vi "SAOMM-OffsetGUI.vi"(0 "Hexapod VRN":refnum<visa-resource-name>="COM4", 1 "Active Refnum":refnum<vi>, 2 "PrAMS-ACK":refnum<vi>, 7 "output cluster":T1, 13 "MessageType":cluster{string[], u32[]}={["emtError", "emtAreYouThere", "emtAcknowledgment", "emtGetClientType", "emtClientType", "emtGetImageExposureTime", "emtSetImageExposureTime", "emtImageExposureTime", "emtGetOptimalExposureTime", "emtSetOptimalExposureTime", "emtOptimalExposureTime", "emtGetImageEMGain", "emtSetImageEMGain", "emtImageEMGain", "emtGetFPGACtrl", "emtSetFPGACtrl", "emtFPGACtrl", "emtGetImageWidth", "emtSetImageWidth", "emtImageWidth", "emtGetImageHeight", "emtSetImageHeight", "emtImageHeight", "emtGetImageBinning", "emtSetImageBinning", "emtImageBinning", "emtGetImageDisplayFrameRate", "emtSetImageDisplayFrameRate", "emtImageDisplayFrameRate", "emtGetROIWidth", "emtSetROIWidth", "emtROIWidth", "emtGetROIHeight", "emtSetROIHeight", "emtROIHeight", "emtGetROIXOffset", "emtSetROIXOffset", "emtROIXOffset", "emtGetROIYOffset", "emtSetROIYOffset", "emtROIYOffset", "emtStartAcquisition", "mtStopAcquisition", "emtAcquisitionStarted", "emtAcquisitionStopped", "emtGetFalconImage", "emtFalconImage"], [1, 2, 3, 4, 5, 1001, 1101, 1201, 1002, 1102, 1202, 1003, 1103, 1203, 1004, 1104, 1204, 1005, 1105, 1205, 1006, 1106, 1206, 1007, 1107, 1207, 1008, 1108, 1208, 1009, 1109, 1209, 1010, 1110, 1210, 1011, 1111, 1211, 1012, 1112, 1212, 1130, 1131, 1150, 1151, 1070, 1270]}) -> (8 "Error":bool)   [LabVIEW 2011]
uses:
  Polymorphics/Num2littleEndian(DBL).vi
panel:
  in  "Signature":u32=1886544237
  in  "Cancel":bool
  in  "Send":bool
  in  "X":dbl caption="Pos" format="%.4f"
  in  "Y":dbl caption="Pos" format="%.4f"
  in  "Z":dbl caption="Pos" format="%.4f"
  in  "U":dbl caption="Pos" format="%.4f"
  in  "V":dbl caption="Pos" format="%.4f"
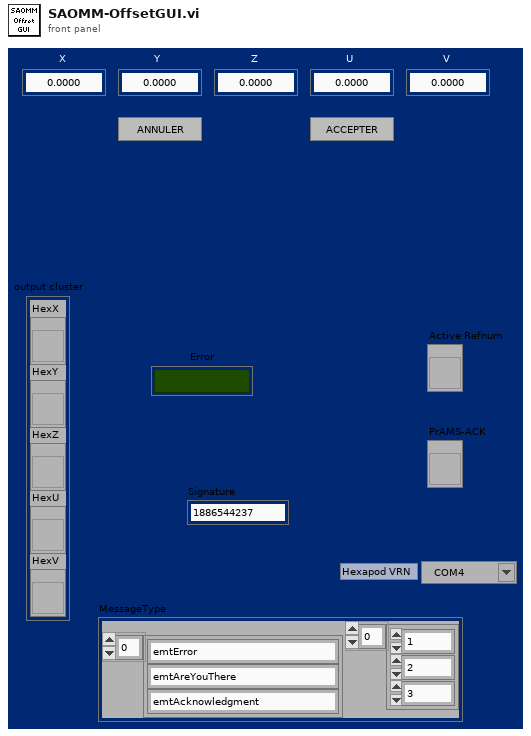
[diagram p1: front panel]
types:
  T1 = cluster{"HexX":refnum<vi>, "HexY":refnum<vi>, "HexZ":refnum<vi>, "HexU":refnum<vi>, "HexV":refnum<vi>}
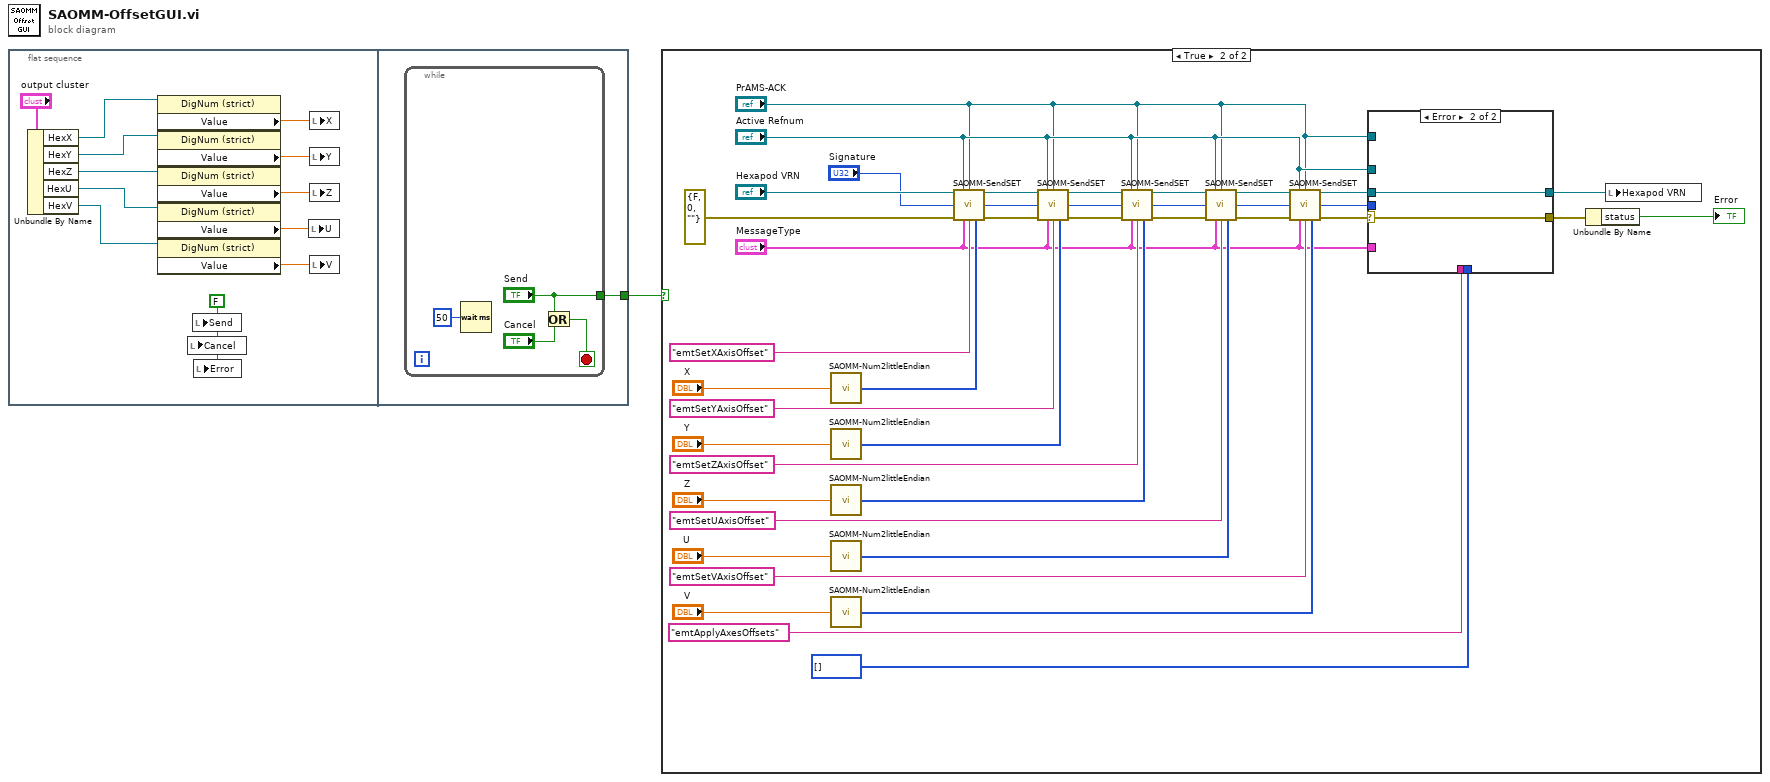
[diagram p0: block diagram]
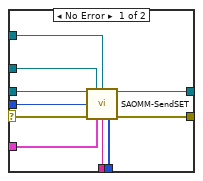
[diagram p3: hidden frame]
diagram:
  n1 = flat-sequence {
    tunnel: [w14] -> w1
    frame #0 {
      w2 = FALSE
      n2 = Unbundle By Name("output cluster") -> ("HexX"=w12:refnum<vi>, "HexY"=w11:refnum<vi>, "HexZ"=w10:refnum<vi>, "HexU"=w9:refnum<vi>, "HexV"=w8:refnum<vi>)
      n3 = property class="DigNum (strict)"(reference=w12) -> ("Value"=w3:dbl)  [unwired: 1 in, 2 out]
      n4 = property class="DigNum (strict)"(reference=w11) -> ("Value"=w4:dbl)  [unwired: 1 in, 2 out]
      n5 = property class="DigNum (strict)"(reference=w10) -> ("Value"=w5:dbl)  [unwired: 1 in, 2 out]
      n6 = property class="DigNum (strict)"(reference=w9) -> ("Value"=w6:dbl)  [unwired: 1 in, 2 out]
      n7 = property class="DigNum (strict)"(reference=w8) -> ("Value"=w7:dbl)  [unwired: 1 in, 2 out]
      n8 = local write "Cancel"(w2) -> ()
      n9 = local write "Send"(w2) -> ()
      n10 = local write "Error"(w2) -> ()
      n11 = local write "U"(w6) -> ()
      n12 = local write "X"(w3) -> ()
      n13 = local write "Y"(w4) -> ()
      n14 = local write "Z"(w5) -> ()
      n15 = local write "V"(w7) -> ()
    }
    frame #1 {
      n16 = while {
        tunnel: ["Send"] -> w14
        stop <- w17 stop-if-true
        n17 = Wait (ms)(milliseconds to wait=u32 50) -> ()  [unwired: 1 out]
        n18 = Or(x="Send", y="Cancel") -> (x .or. y?=w17:bool)
      }
    }
  }
  n19 = case shown="True" w1 {
    frame False {
    }
    frame True {
      n20 = call-poly "SAOMM-Num2littleEndian.vi"("Number"="X") -> ("LiitleEndianedData"=w41:u8[])  [unwired: 14 in]
      n21 = call-poly "SAOMM-Num2littleEndian.vi"("Number"="Y") -> ("LiitleEndianedData"=w42:u8[])  [unwired: 14 in]
      n22 = call-poly "SAOMM-Num2littleEndian.vi"("Number"="Z") -> ("LiitleEndianedData"=w43:u8[])  [unwired: 14 in]
      n23 = call-poly "SAOMM-Num2littleEndian.vi"("Number"="U") -> ("LiitleEndianedData"=w46:u8[])  [unwired: 14 in]
      n24 = call-poly "SAOMM-Num2littleEndian.vi"("Number"="V") -> ("LiitleEndianedData"=w47:u8[])  [unwired: 14 in]
      n25 = call "SAOMM-SendSET.vi"("PRAMMS-COMM IN"="Hexapod VRN", "Active Refnum"="Active Refnum", "PrAMS-ACK"="PrAMS-ACK", "Signature"="Signature", "Error IN"=errorcluster {"status"=FALSE, "code"=0, "source"=""}, "MessageType"="MessageType", "Active SET"="emtSetXAxisOffset", "Value (little endianed byte array)"=w41) -> ("PRAMMS-COMM OUT"=w32:refnum<visa-resource-name>, "Error OUT"=w38:errorcluster)  [unwired: 4 in, 2 out]
      n26 = call "SAOMM-SendSET.vi"("PRAMMS-COMM IN"=w32, "Active Refnum"="Active Refnum", "PrAMS-ACK"="PrAMS-ACK", "Signature"="Signature", "Error IN"=w38, "MessageType"="MessageType", "Active SET"="emtSetYAxisOffset", "Value (little endianed byte array)"=w42) -> ("PRAMMS-COMM OUT"=w33:refnum<visa-resource-name>, "Error OUT"=w37:errorcluster)  [unwired: 4 in, 2 out]
      n27 = call "SAOMM-SendSET.vi"("PRAMMS-COMM IN"=w33, "Active Refnum"="Active Refnum", "PrAMS-ACK"="PrAMS-ACK", "Signature"="Signature", "Error IN"=w37, "MessageType"="MessageType", "Active SET"="emtSetZAxisOffset", "Value (little endianed byte array)"=w43) -> ("PRAMMS-COMM OUT"=w53:refnum<visa-resource-name>, "Error OUT"=w36:errorcluster)  [unwired: 4 in, 2 out]
      n28 = call "SAOMM-SendSET.vi"("PRAMMS-COMM IN"=w53, "Active Refnum"="Active Refnum", "PrAMS-ACK"="PrAMS-ACK", "Signature"="Signature", "Error IN"=w36, "MessageType"="MessageType", "Active SET"="emtSetUAxisOffset", "Value (little endianed byte array)"=w46) -> ("PRAMMS-COMM OUT"=w54:refnum<visa-resource-name>, "Error OUT"=w35:errorcluster)  [unwired: 4 in, 2 out]
      n29 = call "SAOMM-SendSET.vi"("PRAMMS-COMM IN"=w54, "Active Refnum"="Active Refnum", "PrAMS-ACK"="PrAMS-ACK", "Signature"="Signature", "Error IN"=w35, "MessageType"="MessageType", "Active SET"="emtSetVAxisOffset", "Value (little endianed byte array)"=w47) -> ("PRAMMS-COMM OUT"=w52:refnum<visa-resource-name>, "Error OUT"=w51:errorcluster)  [unwired: 4 in, 2 out]
      n30 = case shown="Error" w51 {
        selector: w51 -> [w56 w65]
        tunnel: "Active Refnum" -> [w64 _]
        tunnel: "PrAMS-ACK" -> [w63 _]
        tunnel: "Signature" -> [w62 _]
        tunnel: [w61 w66] -> w34
        tunnel: [w60 w65] -> w20
        tunnel: "MessageType" -> [w59 _]
        tunnel: "emtApplyAxesOffsets" -> [w58 _]
        tunnel: u8[] [] ("Value (little endianed byte array)") -> [w57 _]
        tunnel: w52 -> [w55 w66]
        frame No Error {
          n31 = call "SAOMM-SendSET.vi"("PRAMMS-COMM IN"=w55, "Active Refnum"=w64, "PrAMS-ACK"=w63, "Signature"=w62, "Error IN"=w56, "MessageType"=w59, "Active SET"=w58, "Value (little endianed byte array)"=w57) -> ("PRAMMS-COMM OUT"=w61:refnum<visa-resource-name>, "Error OUT"=w60:errorcluster)  [unwired: 4 in, 2 out]
        }
        frame Error {
        }
      }
      n32 = Unbundle By Name(w20) -> ("status"=→"Error":bool)
      n33 = local write "Hexapod VRN"(w34) -> ()
    }
  }
